vi "veristandSteps-installer-update.vi"   [LabVIEW 2014, in "veristand-steps-build-system.lvlib"]
uses:
  veristand-steps-build-system.lvlib
  <vilib>/Wiresmith Technology/LabVIEW CLI/CLI Class/CLI.lvclass
types:
  T1 = typedef "veristand-steps-build-system.lvlib/LVInstallerMutationSession.ctl" = cluster{"Installer Build Specification Ref":refnum<vi>, "Project reference out":refnum<vi>, "Installer Project Path":path}
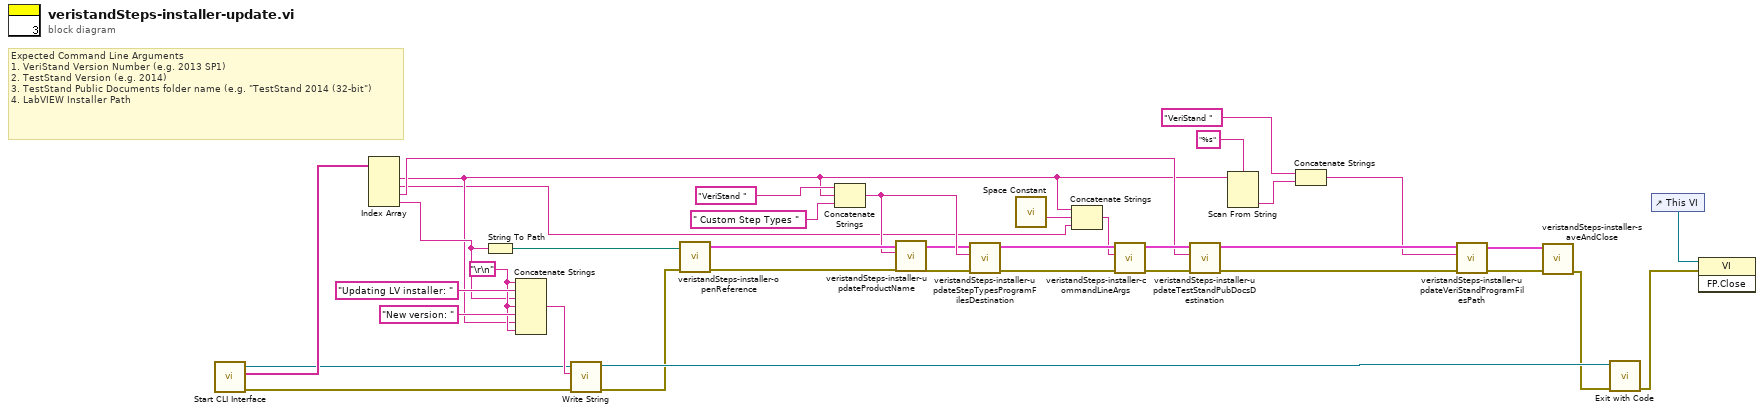
[diagram p0: block diagram]
diagram:
  w24 = "\r\n"
  # "Expected Command Line Arguments\n1. VeriStand Version Number (e.g. 2013 SP1)\n2. TestStand Version (e.g. 2014)\n3. TestStand Public Documents folder name (e.g. \"TestStand 2014 (32-bit\")\n4. LabVIEW Installer Path"
  n1 = call <vilib>:"Start CLI Interface.vi"() -> ("error out"=w27:errorcluster, "Custom Parameters"=w28:string[], "CLI out"=w22:refnum<class "CLI.lvclass">)  [unwired: 9 in]
  n2 = Index Array(array=w28) -> (element #1=w4:string, element #2=w2:string, element #3=w5:string, element #4=w6:string)  [unwired: 4 in]
  n3 = String To Path(string=w6) -> (path=w35:path)
  n4 = Concatenate Strings(w24, "Updating LV installer: " ("string"), w6, w24, "New version: " ("string"), w4, w24) -> (w23:string)
  n5 = call <vilib>:"Write String.vi"("error in (no error)"=w27, "Text to Write"=w23, "CLI in"=w22) -> ("error out"=w19:errorcluster, "CLI out"=w20:refnum<class "CLI.lvclass">)  [unwired: 7 in]
  n6 = call "veristandSteps-installer-openReference.vi"("error in (no error)"=w19, "Installer Project Path"=w35) -> ("error out"=w18:errorcluster, "InstallerSession"=w34:T1)  [unwired: 8 in]
  n7 = Concatenate Strings("VeriStand " ("string"), w4, " Custom Step Types " ("string")) -> (w32:string)
  n8 = call "veristandSteps-installer-updateProductName.vi"("error in (no error)"=w18, "Installer Product Name"=w32, "InstallerMutationSession"=w34) -> ("error out"=w33:errorcluster, "InstallerMutationSession out"=w31:T1)  [unwired: 7 in]
  n9 = call "veristandSteps-installer-updateStepTypesProgramFilesDestination.vi"("error in (no error)"=w33, "New Application Directory Name"=w32, "InstallerMutationSession"=w31) -> ("error out"=w30:errorcluster, "InstallerMutationSession out"=w29:T1)  [unwired: 7 in]
  n10 = call <vilib>:"Space Constant.vi"() -> ("String"=w3:string)
  n11 = Concatenate Strings(w4, w3, w2) -> (w1:string)
  n12 = call "veristandSteps-installer-commandLineArgs.vi"("error in (no error)"=w30, "New Command Line Argument(s)"=w1, "InstallerMutationSession"=w29) -> ("error out"=w17:errorcluster, "InstallerMutationSession out"=w16:T1)  [unwired: 7 in]
  n13 = call "veristandSteps-installer-updateTestStandPubDocsDestination.vi"("error in (no error)"=w17, "TestStand Public Docs Folder Name"=w5, "InstallerMutationSession"=w16) -> ("error out"=w14:errorcluster, "InstallerMutationSession out"=w8:T1)  [unwired: 7 in]
  n14 = Scan From String(format string="%s", input string=w4) -> (output 1=w9:string)  [unwired: 3 in, 3 out]
  n15 = Concatenate Strings("VeriStand " ("string"), w9) -> (w7:string)
  n16 = call "veristandSteps-installer-updateVeriStandProgramFilesPath.vi"("error in (no error)"=w14, "VeriStand Applicatin Program Files Directroy"=w7, "InstallerMutationSession"=w8) -> ("error out"=w13:errorcluster, "InstallerMutationSession out"=w12:T1)  [unwired: 7 in]
  n17 = call "veristandSteps-installer-saveAndClose.vi"("error in (no error)"=w13, "InstallerMutationSession"=w12) -> ("error out"=w15:errorcluster)  [unwired: 9 in]
  n18 = call <vilib>:"Exit with Code.vi"("error in (no error)"=w15, "CLI in"=w20) -> ("error out"=w21:errorcluster)  [unwired: 9 in]
  n19 = control-ref of="This VI"() -> (w36:refnum<vi>)
  n20 = invoke class="VI" method="FP.Close"(reference=w36, error in=w21) -> ()  [unwired: 1 in, 3 out]
